vi "ProduceLiveImages.vi"(6 "Max Images In":T1, 7 "Laser Mode":string, 8 "error IO":errorcluster, 9 "Images In":T3[](array[typedef]), 10 "LUT in":T2 {"LUT Red Max" scale=0.8..10000.0; "LUT Green Max" scale=0.8..40000.0}, 11 "Image Data IN":cluster{u16[], u16[], i32, i32}) -> (0 "error out":errorcluster, 1 "Images Out":T3[](array[typedef]), 2 "LUT out":T2, 4 "Max Images Out":T1)   [LabVIEW 2015]
uses:
  <vilib>/vision/Image Controls.llb/IMAQ Image.ctl
  LiveImage_Global.vi
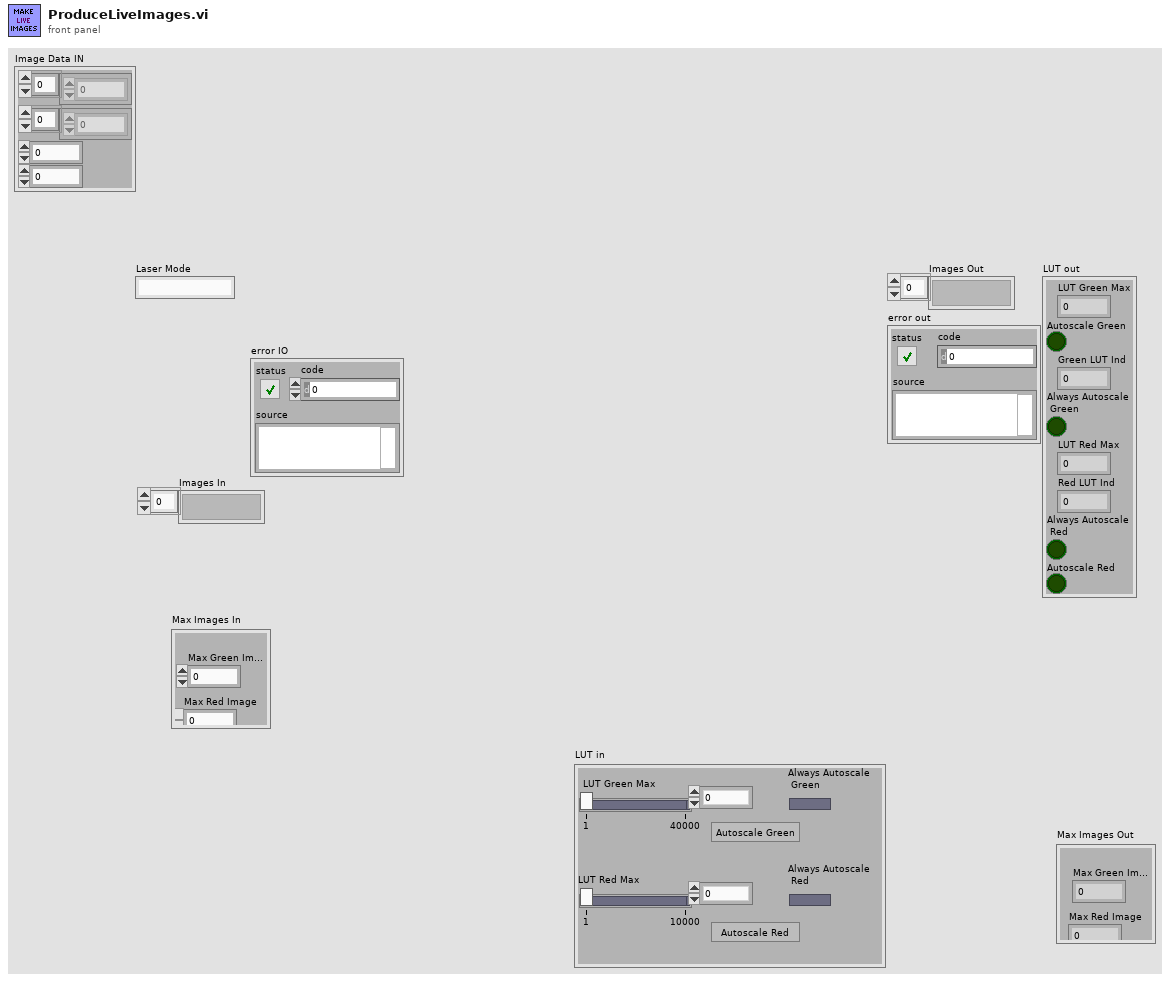
[diagram p1: front panel]
types:
  T1 = cluster{"Max Green Image":u16, "Max Red Image":u16}
  T2 = cluster{"LUT Green Max":u16, "Autoscale Green":bool, "Green LUT Ind":u16, "Always Autoscale\n Green":bool, "LUT Red Max":u16, "Red LUT Ind":u16, "Always Autoscale\n Red":bool, "Autoscale Red":bool}
  T3 = typedef "IMAQ Image.ctl" = refnum<image>
  T4 = cluster{"element":u16, "element":u16, u16, "n":u16}[]
  T5 = cluster{"element":u16, "element":u16, u16, "n":u16}[][]
  T6 = cluster{"element":u16, u16, "element":u16, i32}[]
  T7 = cluster{"element":u16, u16, "element":u16, i32}[][]
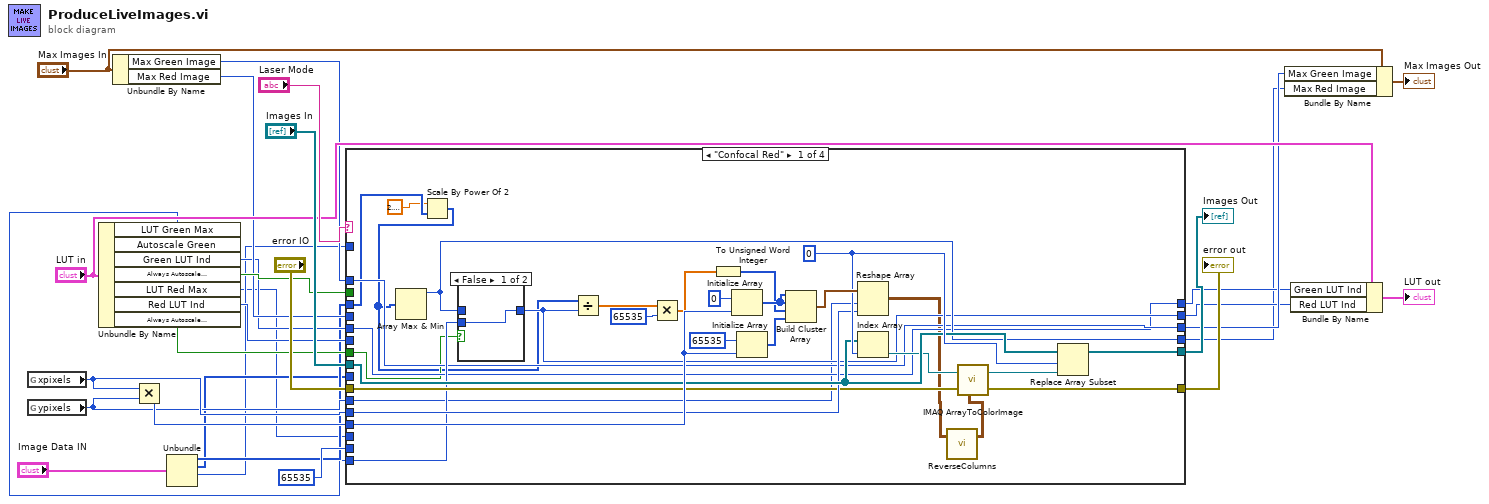
[diagram p0: block diagram]
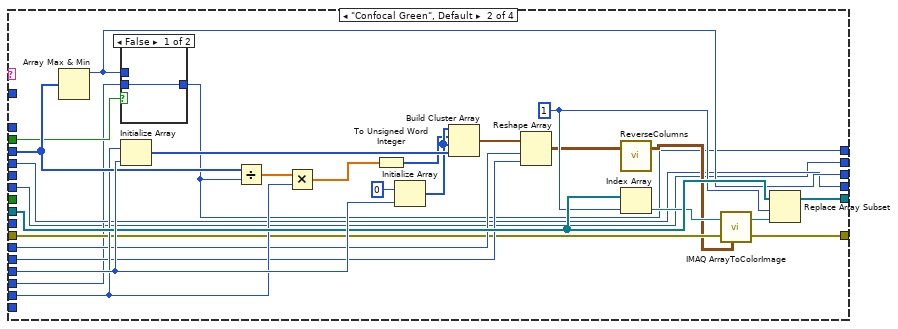
[diagram p3: hidden frame]
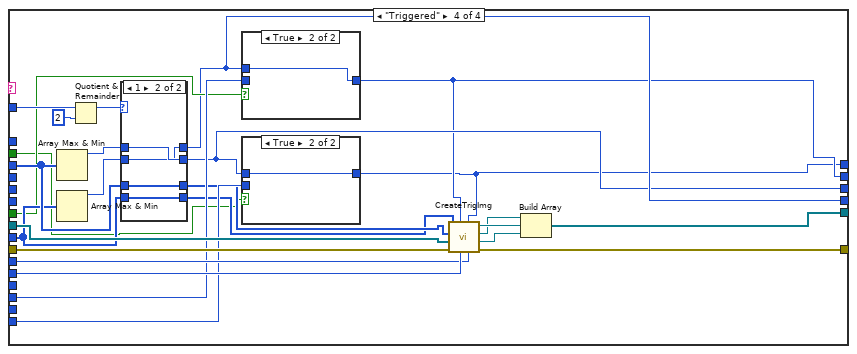
[diagram p6: hidden frame]
diagram:
  n1 = global read "LiveImage_Global.vi" "xpixels"() -> (w28:i32)
  n2 = global read "LiveImage_Global.vi" "ypixels"() -> (w26:i32)
  n3 = Unbundle By Name("LUT in") -> ("LUT Green Max"=w1:u16, "Green LUT Ind"=w9:u16, "Always Autoscale\n Green"=w20:bool, "LUT Red Max"=w2:u16, "Red LUT Ind"=w10:u16, "Always Autoscale\n Red"=w19:bool)  [unwired: 1 out]
  n4 = Unbundle By Name("Max Images In") -> ("Max Green Image"=w16:u16, "Max Red Image"=w15:u16)
  n5 = Multiply(x=w28, y=w26) -> (x*y=w27:i32)
  n6 = Unbundle("Image Data IN") -> (w7:u16[], w6:u16[], w5:i32)  [unwired: 1 out]
  n7 = case shown="\"Confocal Red\"" "Laser Mode" {
    tunnel: w7 -> [w31 w77 _ w108]
    tunnel: w5 -> [_ _ _ w122]
    tunnel: "Images In" -> [w54 w84 w96 w120]
    tunnel: w28 -> [w46 w72 _ w119]
    tunnel: [w53 w82 w96 w118] -> w25
    tunnel: w27 -> [w57 w86 _ _]
    tunnel: w26 -> [w35 w73 _ w115]
    tunnel: 65535 -> [_ w76 _ _]
    tunnel: "error IO" -> [w45 w71 w95 w117]
    tunnel: [w44 w70 w95 w116] -> w23
    tunnel: w6 -> [_ _ _ w107]
    tunnel: w20 -> [_ w67 _ w101]
    tunnel: w19 -> [w36 _ _ w102]
    tunnel: w1 -> [w41 _ _ w114]
    tunnel: w2 -> [_ w64 _ w113]
    tunnel: w16 -> [w39 _ w94 _]
    tunnel: w15 -> [_ w65 w93 _]
    tunnel: [w40 w65 w93 w100] -> w3
    tunnel: [w39 w66 w94 w99] -> w12
    tunnel: [w38 w62 w91 w98] -> w11
    tunnel: w10 -> [_ w62 w91 _]
    tunnel: w9 -> [w37 _ w92 _]
    tunnel: [w37 w63 w92 w97] -> w8
    frame "Confocal Red" {
      w55 = 0 ("index")
      n8 = Scale By Power Of 2(n=2.718281828459045, x=w31) -> (x*2^n=w32:u16[])
      n9 = Array Max & Min(array=w32) -> (max value=w40:u16)  [unwired: 3 out]
      n10 = case shown="False" w36 {
        tunnel: w40 -> [_ w61]
        tunnel: [w60 w61] -> w38
        tunnel: w41 -> [w60 _]
        frame False {
        }
        frame True {
        }
      }
      n11 = Divide(x=w32, y=w38) -> (x/y=w48:dbl[])
      n12 = Multiply(x=w48, y=65535) -> (x*y=w49:dbl[])
      n13 = To Unsigned Word Integer(number=w49) -> (unsigned 16bit integer=w47:u16[])
      n14 = Initialize Array(u16 0 ("element"), w57) -> (w56:u16[])
      n15 = Initialize Array(u16 65535 ("n"), w57) -> (w43:u16[])
      n16 = Build Cluster Array(w56, w56, w47, w43) -> (w59:T4)
      n17 = Reshape Array(w59, w35, w46) -> (w34:T5)
      n18 = Index Array(array=w54, index=w55) -> (element=w52:T3)
      n19 = call "ReverseColumns.vi"("output array 2"=w34) -> ("transposed array"=w33:T5)  [unwired: 2 in]
      n20 = call "IMAQ ArrayToColorImage"("Image"=w52, "Image Pixels (U64)"=w33, "error in (no error)"=w45) -> ("Image Out"=w42:T3, "error out"=w44:errorcluster)  [unwired: 2 in]
      n21 = Replace Array Subset(array=w54, new element=w42, index=w55) -> (w53:T3[])
    }
    frame "Confocal Green", Default {
      w74 = 1 ("index")
      n22 = Array Max & Min(array=w77) -> (max value=w66:u16)  [unwired: 3 out]
      n23 = case shown="False" w67 {
        tunnel: w66 -> [_ w90]
        tunnel: [w89 w90] -> w63
        tunnel: w64 -> [w89 _]
        frame False {
        }
        frame True {
        }
      }
      n24 = Initialize Array(w76, w86) -> (w85:i32[])
      n25 = Divide(x=w77, y=w63) -> (x/y=w79:dbl[])
      n26 = Multiply(x=w79, y=w76) -> (x*y=w78:dbl[])
      n27 = To Unsigned Word Integer(number=w78) -> (unsigned 16bit integer=w75:u16[])
      n28 = Initialize Array(u16 0 ("element"), w86) -> (w80:u16[])
      n29 = Build Cluster Array(w80, w75, w80, w85) -> (w88:T6)
      n30 = Reshape Array(w88, w73, w72) -> (w69:T7)
      n31 = call "ReverseColumns.vi"("output array 2"=w69) -> ("transposed array"=w68:T5)  [unwired: 2 in]
      n32 = Index Array(array=w84, index=w74) -> (element=w83:T3)
      n33 = call "IMAQ ArrayToColorImage"("Image"=w83, "Image Pixels (U64)"=w68, "error in (no error)"=w71) -> ("Image Out"=w81:T3, "error out"=w70:errorcluster)  [unwired: 2 in]
      n34 = Replace Array Subset(array=w84, new element=w81, index=w74) -> (w82:T3[])
    }
    frame "Confocal Blue" {
    }
    frame "Triggered" {
      n35 = Array Max & Min(array=w108) -> (max value=w106:u16)  [unwired: 3 out]
      n36 = Array Max & Min(array=w107) -> (max value=w105:u16)  [unwired: 3 out]
      n37 = Quotient & Remainder(x=w122, y=2) -> (x-y*floor(x/y)=w109:i32)  [unwired: 1 out]
      n38 = case shown="1" w109 {
        tunnel: w108 -> [w125 w130]
        tunnel: [w126 w130] -> w104
        tunnel: w107 -> [w126 w129]
        tunnel: [w125 w129] -> w103
        tunnel: w105 -> [w123 w127]
        tunnel: w106 -> [w124 w128]
        tunnel: [w123 w128] -> w99
        tunnel: [w124 w127] -> w100
        frame 0, Default {
        }
        frame 1 {
        }
      }
      n39 = case shown="True" w102 {
        tunnel: [w133 w134] -> w98
        tunnel: w100 -> [_ w134]
        tunnel: w113 -> [w133 _]
        frame False {
        }
        frame True {
        }
      }
      n40 = case shown="True" w101 {
        tunnel: [w131 w132] -> w97
        tunnel: w114 -> [w131 _]
        tunnel: w99 -> [_ w132]
        frame False {
        }
        frame True {
        }
      }
      n41 = call "CreateTrigImg.vi"("Y Pixels"=w115, "Max Green"=w97, "X Pixels"=w119, "Max Red"=w98, "error in (no error)"=w117, "Images In"=w120, "Green Data"=w104, "Red Data"=w103) -> ("error out"=w116:errorcluster, "Trig Img Out"=w110:T3, "Red Image Out"=w111:T3, "Green Image Out"=w112:T3)
      n42 = Build Array(w111, w112, w110) -> (w118:T3[])
    }
  }
  "Images Out" <- w25
  "error out" <- w23
  n43 = Bundle By Name(cluster="Max Images In", "Max Green Image"=w12, "Max Red Image"=w3) -> (→"Max Images Out":T1)
  n44 = Bundle By Name(cluster="LUT in", "Green LUT Ind"=w8, "Red LUT Ind"=w11) -> (→"LUT out":T2)
